vi "pop_thread.vi"(8 "error in (no error)":errorcluster, 11 "Lua in":refnum<class "Lua.lvclass">) -> (0 "error out":errorcluster, 2 "Thread":refnum<class "Lua Thread.lvclass">, 3 "Lua out":refnum<class "Lua.lvclass">)   [LabVIEW 2020, in "Lua for LabVIEW.lvlib" / "Lua.lvclass"]
doc: "Pop a numeric value from the stack."
uses:
  Lua.lvclass
  Lua Thread/Lua Thread.lvclass
  Lua.lvclass/Lua.ctl
  lib/lua.dll/lua_settop.vi
  lib/lua.dll/lua.dll.lvlib
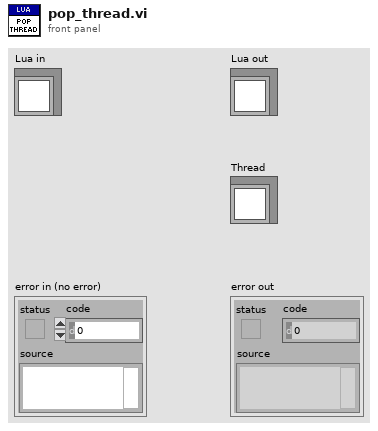
[diagram p1: front panel]
types:
  T1 = typedef "lua.dll.lvlib/lua_types.ctl" = i32
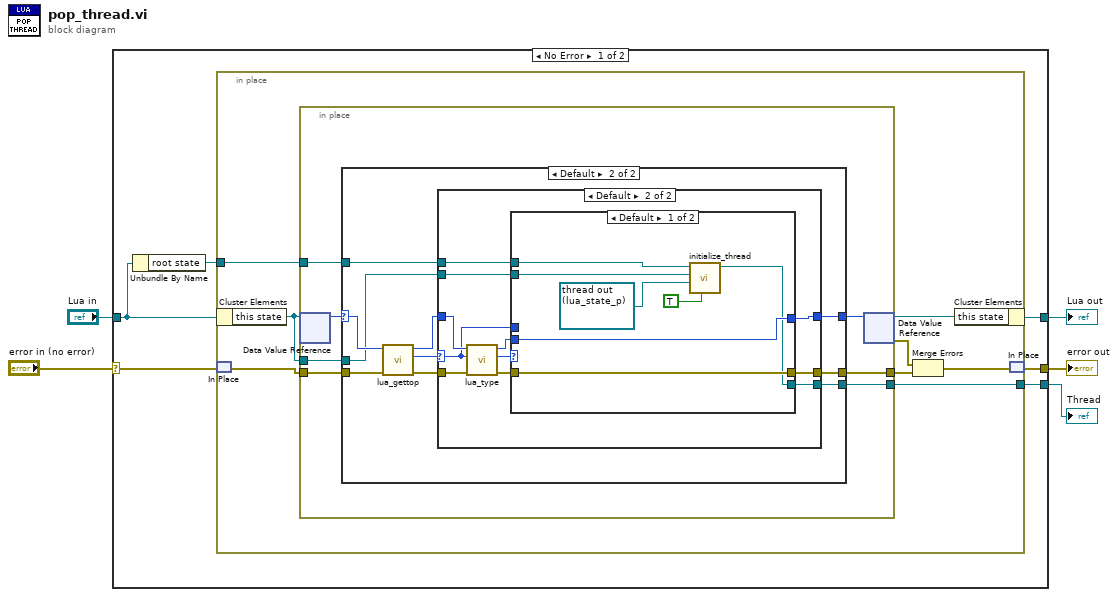
[diagram p0: block diagram]
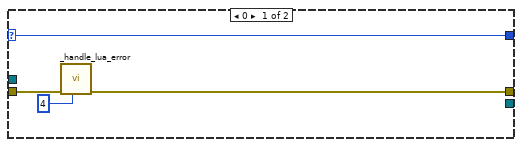
[diagram p2: hidden frame]
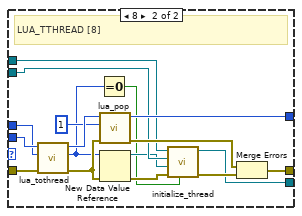
[diagram p4: hidden frame]
diagram:
  n1 = case shown="No Error" "error in (no error)" {
    selector: "error in (no error)" -> [w9 w79]
    tunnel: [w10 w79] -> w2
    tunnel: [w11 w78] -> w3
    tunnel: "Lua in" -> [w7 w78]
    tunnel: [w8 _] -> w1
    frame No Error {
      n2 = Unbundle By Name(w7) -> ("root state"=w6:refnum<data-value>)
      n3 = in-place {
        in-place-border: [w18] -> w8
        in-place-border: w6 -> [w12]
        n4 = in-place-cluster #1(w7) -> ("this state"=w17:refnum<data-value>)
        n5 = in-place-match #2(w9) -> (w19:errorcluster)
        n6 = in-place {
          in-place-border: w19 -> [w26]
          in-place-border: [w25] -> w14
          in-place-border: [w24] -> w18
          in-place-border: w17 -> [w23]
          in-place-border: w12 -> [w20]
          n7 = in-place-dvr #3(w17) -> (w22:u64)  [unwired: 1 out]
          n8 = case shown="Default" w22 {
            selector: w22 -> [w30 w37]
            tunnel: [w30 w40] -> w21
            tunnel: w26 -> [w27 w38]
            tunnel: [w28 w39] -> w25
            tunnel: w23 -> [_ w33]
            tunnel: [_ w32] -> w24
            tunnel: w20 -> [_ w31]
            frame 0 {
              n9 = call "_handle_lua_error.vi"("lua status"=4 ("lua_load errcode"), "error in (no error)"=w27) -> ("error out"=w28:errorcluster)  [unwired: 9 in]
            }
            frame Default {
              n10 = call "lua_gettop.vi"("error in (no error)"=w38, "lua_state_p"=w37) -> ("error out"=w35:errorcluster, "index"=w34:i32, "lua_state_p out"=w36:u64)  [unwired: 7 in]
              n11 = case shown="Default" w34 {
                selector: w34 -> [_ w48]
                tunnel: [w42 w47] -> w40
                tunnel: [w41 w46] -> w39
                tunnel: w36 -> [w42 w50]
                tunnel: w35 -> [w41 w49]
                tunnel: w33 -> [_ w45]
                tunnel: [_ w44] -> w32
                tunnel: w31 -> [_ w43]
                frame 0 {
                }
                frame Default {
                  n12 = call "lua_type.vi"("error in (no error)"=w49, "index"=w48, "lua_state_p"=w50) -> ("error out"=w51:errorcluster, "lua type"=w53:T1, "lua_state_p out"=w52:u64)  [unwired: 6 in]
                  n13 = case shown="Default" w53 {
                    tunnel: [w59 w72] -> w47
                    tunnel: w52 -> [w59 w77]
                    tunnel: [w60 w69] -> w46
                    tunnel: w51 -> [w60 w75]
                    tunnel: w48 -> [_ w76]
                    tunnel: w45 -> [w57 w65]
                    tunnel: [w54 w66] -> w44
                    tunnel: w43 -> [w58 w63]
                    frame Default {
                      n14 = call "initialize_thread.vi"("done?"=TRUE, "this state"=refnum<data-value> refnum, "parent state"=w57, "root state"=w58) -> ("Lua for LabVIEW.lvlib:Lua Thread.lvclass"=w54:refnum<class "Lua Thread.lvclass">)  [unwired: 6 in, 1 out]
                    }
                    frame 8 {
                      # "LUA_TTHREAD [8]"
                      n15 = call "lua_tothread.vi"("error in (no error)"=w75, "index"=w76, "lua_state_p"=w77) -> ("error out"=w71:errorcluster, "thread out (lua_state_p)"=w62:u64, "lua_state_p out"=w74:u64)  [unwired: 6 in]
                      n16 = Equal To 0?(x=w62) -> (x = 0?=w61:bool)
                      n17 = call "lua_pop.vi"("error in (no error)"=w71, "n"=1, "lua_state_p"=w74) -> ("error out"=w70:errorcluster, "lua_state_p out"=w72:u64)  [unwired: 7 in]
                      n18 = New Data Value Reference(data value=w62, error in=w71) -> (data value reference=w64:refnum<data-value>, error out=w68:errorcluster)
                      n19 = call "initialize_thread.vi"("done?"=w61, "error in"=w68, "this state"=w64, "parent state"=w65, "root state"=w63) -> ("error out"=w67:errorcluster, "Lua for LabVIEW.lvlib:Lua Thread.lvclass"=w66:refnum<class "Lua Thread.lvclass">)  [unwired: 5 in]
                      n20 = Merge Errors(w70, w67) -> (w69:errorcluster)
                    }
                  }
                }
              }
            }
          }
          n21 = in-place-dvr #3(w21) -> (w16:refnum<data-value>, w15:errorcluster)
        }
        n22 = Merge Errors(w15, w14) -> (w13:errorcluster)
        n23 = in-place-cluster #1("this state"=w16) -> (w11:refnum<class "Lua.lvclass">)
        n24 = in-place-match #2(w13) -> (w10:errorcluster)
      }
    }
    frame Error {
    }
  }
  "error out" <- w2
  "Lua out" <- w3
  "Thread" <- w1
